vi "SSL Vision Log Player.vi"() -> ()   [LabVIEW 2016]
uses:
  SSL Detection Frame.ctl
  SSL Detection Robot.ctl
  SSL Detection Ball.ctl
  <extravilib>/ChannelInstances/Stream-a[.](u8)/Read With Abort.vi
  <extravilib>/ChannelInstances/Stream-a[.](u8)/Write With Abort.vi
  <extravilib>/ChannelInstances/Stream-a[.](u8)/Endpoint.vi
  <vilib>/Utility/tcp.llb/UDP Multicast Read-Only Open.vi
  <extravilib>/ChannelInstances/Stream-a[.](u8)/Instantiate.vi
  <extravilib>/ChannelInstances/Stream-a[.](u8)/)Channel.vi
  <resource>/ChannelSupport/_ChannelSupport/WaitIfNeeded.vi
  Varint Decoder uint64.vi
  Varint Decoder uint32.vi
  <extravilib>/ChannelInstances/Stream-a[.](u8).lvlib
panel:
  out "Varint 6":u64
  out "Varint 5":u32
  out "Varint 4":u64
  out "Varint 3":i32
  out "Varint 2":u64
  out "Varint":u64
  out "error out 3":errorcluster
  out "Boolean":bool
  out "Boolean 2":bool
  out "error out":errorcluster
  out "count 2":i32
  out "count":i32
  out "2D Picture":picture
  out "Detection Frame 2":T1 {"t_sent" format="%#_6f"; "t_capture" format="%#.6f"}
  in  "Modo":bool
  in  "Multicast Port:":u16=10020
  out "Data Read":i32 format="%.3p"
  out "Numeric":i32
  out "error out 2":errorcluster
  in  "file path (use dialog)":path=path "E:/Media/2016-07-01_cmdragons_immortals.log"
  in  "Multicast Address:":string="224.5.23.2"
  # "UDP"
  # "LOG"
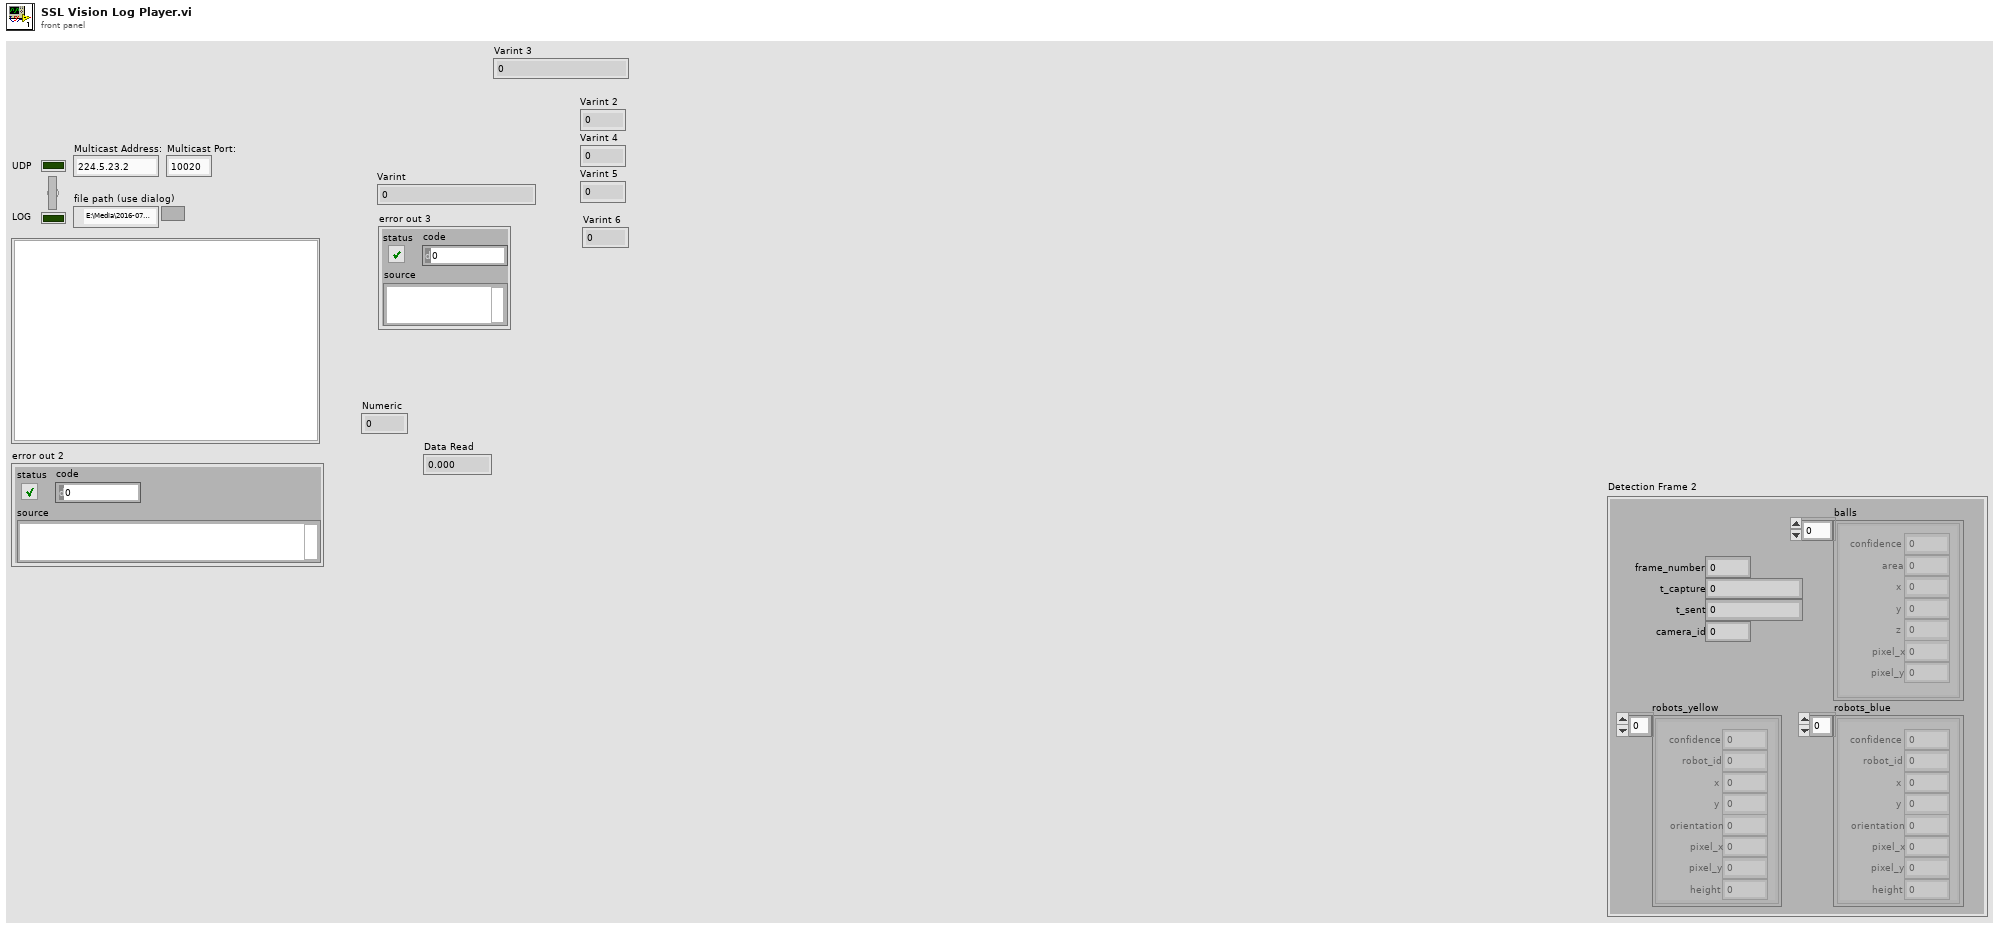
[diagram p1: front panel]
types:
  T1 = typedef "SSL Detection Frame.ctl" = cluster{"frame_number":u32, "t_capture":dbl, "t_sent":dbl, "camera_id":u32, "robots_yellow":T2[], "robots_blue":T2[], "balls":T3[]}
  T2 = typedef "SSL Detection Robot.ctl" = cluster{"x":dbl, "robot_id":u32, "confidence":sgl, "y":sgl, "orientation":sgl, "pixel_x":sgl, "pixel_y":sgl, "height":sgl}
  T3 = typedef "SSL Detection Ball.ctl" = cluster{"x":sgl, "area":u32, "confidence":sgl, "y":sgl, "z":sgl, "pixel_x":sgl, "pixel_y":sgl}
  T4 = enum16{"open", "replace", "create", "open or create", "replace or create", "replace or create with confirmation"}
  T5 = typedef "Stream-a[.](u8).lvlib/)Channel.ctl" = refnum<queue>
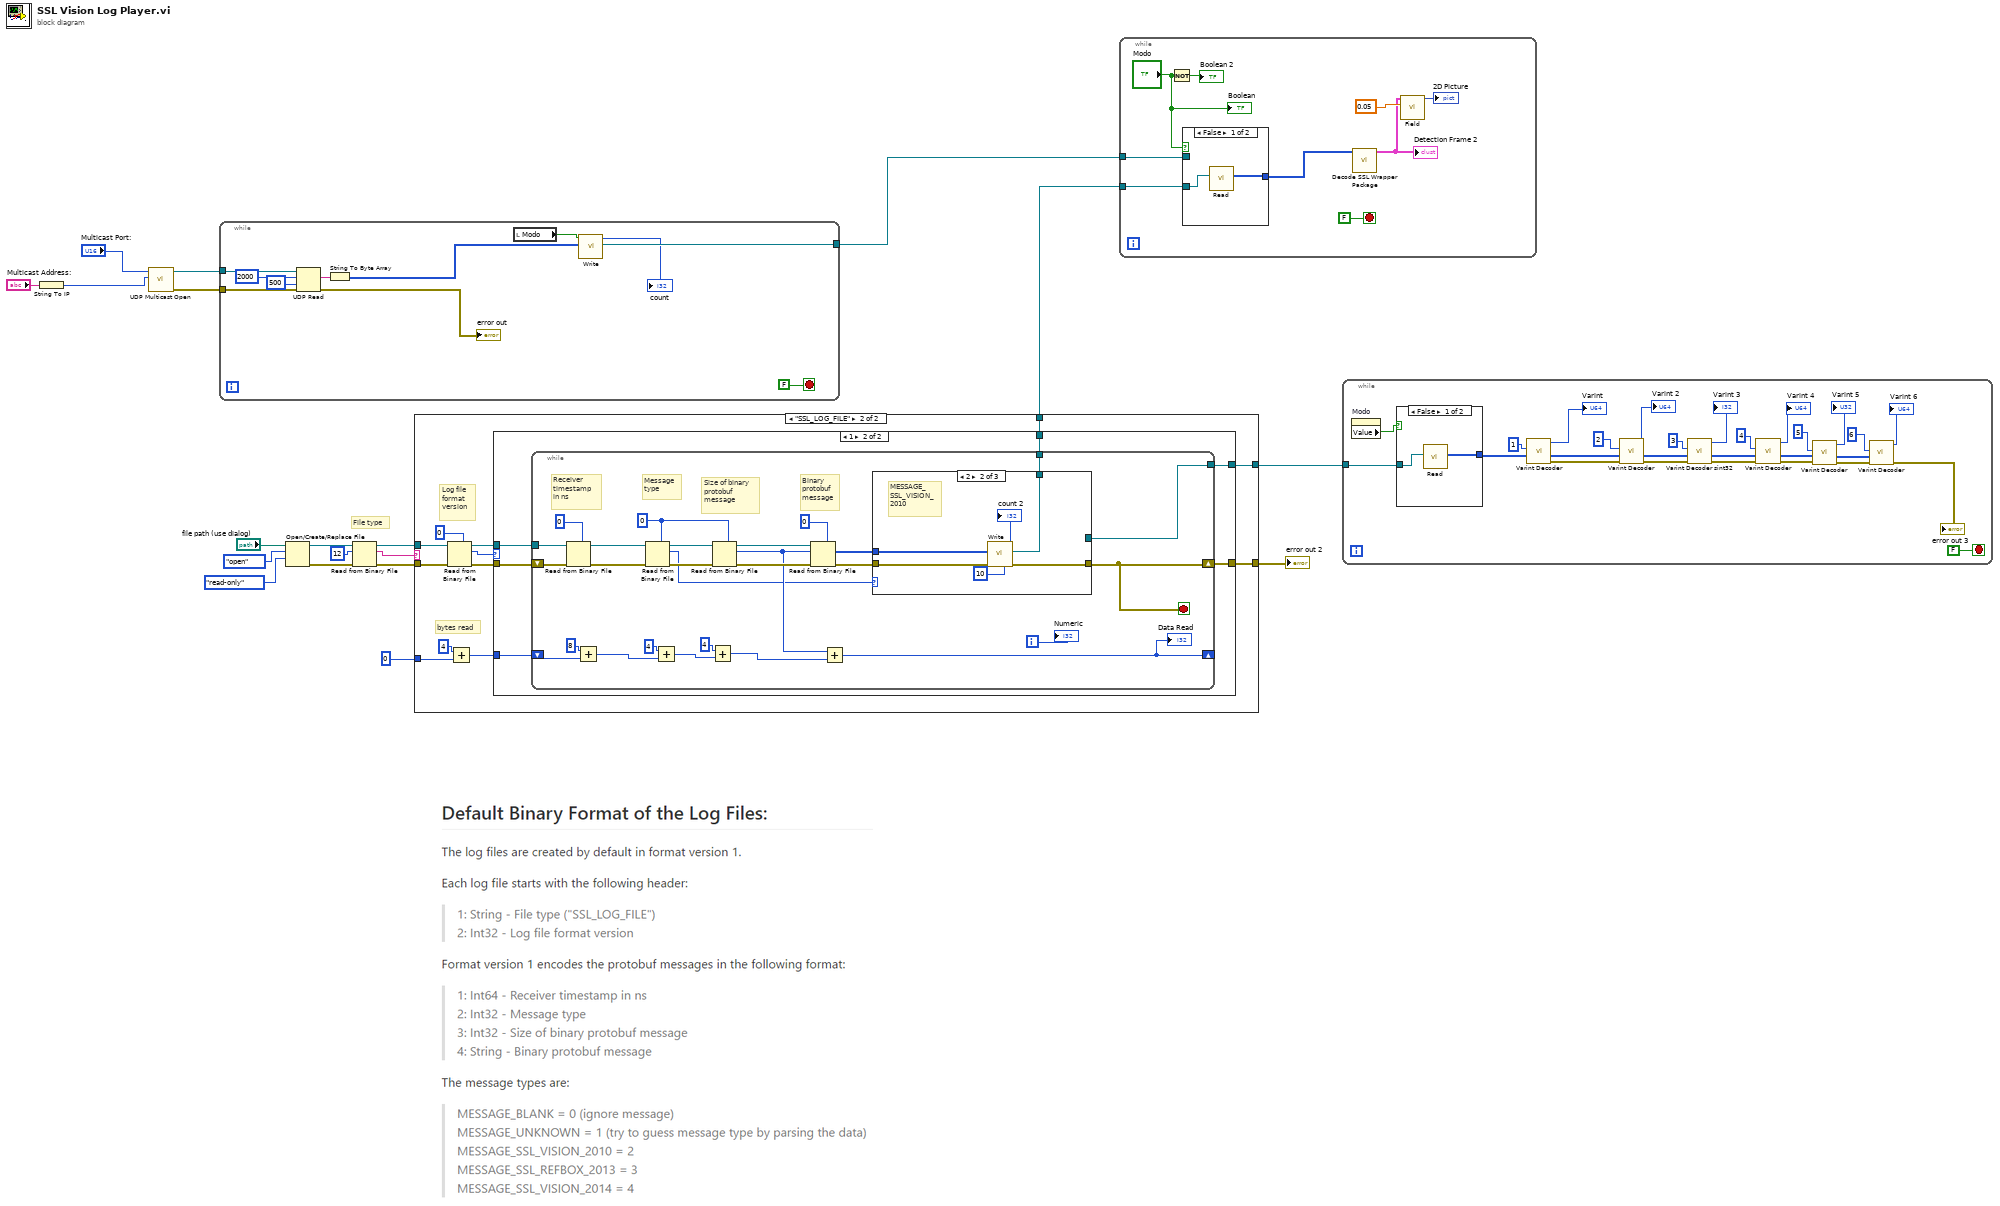
[diagram p0: block diagram]
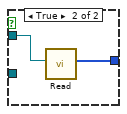
[diagram p3: hidden frame]
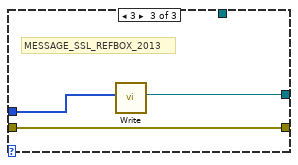
[diagram p7: hidden frame]
diagram:
  # "File type"
  n1 = String To IP(1:"Multicast Address:") -> (0:w18:u32)
  n2 = call-poly <vilib>:"UDP Multicast Open.vi"("multicast addr"=w18, "port"="Multicast Port:") -> ("error out"=w17:errorcluster, "connection ID"=w16:refnum<k16>)  [unwired: 7 in, 1 out]
  n3 = while {
    tunnel: w17 -> [w30]
    tunnel: w16 -> [w29]
    tunnel: [w24] -> w2
    stop <- FALSE stop-if-true
    n4 = UDP Read(connection ID=w29, max size (548)=2000, timeout ms (25000)=500, 8:w30) -> (data out=w28:string, error out=→"error out":errorcluster)  [unwired: 3 out]
    n5 = String To Byte Array(string=w28) -> (unsigned byte array=w25:u8[])
    n6 = local read "Modo"() -> (w21:bool)
    n7 = call <extravilib>:"Write.vi"("element"=w25, "element valid? (T)"=w21) -> ("channel"=w24:T5, "count"=→"count":i32)  [unwired: 7 in, 1 out]
  }
  n8 = Open/Create/Replace File(file path (use dialog)="file path (use dialog)", operation (0:open)=T4."open", access (0:read/write)=enum16{"read/write", "read-only", "write-only"}."read-only") -> (refnum out=w12:refnum<file>, error out=w13:errorcluster)  [unwired: 3 in, 1 out]
  n9 = Read from Binary File(8:w13, 10:12 ("count (1)"), 11:w12) -> (0:w9:errorcluster, 2:w7:string, 3:w10:refnum<file>)  [unwired: 3 in, 1 out]
  n10 = case shown="\"SSL_LOG_FILE\"" w7 {
    tunnel: w10 -> [_ w42]
    tunnel: w9 -> [w31 w41]
    tunnel: 0 -> [_ w38]
    tunnel: [w31 w34] -> w6
    tunnel: [_ w33] -> w3
    tunnel: [_ w32] -> w1
    frame Default {
    }
    frame "SSL_LOG_FILE" {
      # "bytes read"
      # "Log file \nformat \nversion"
      n11 = Read from Binary File(5:0 ("prompt (Open existing file)"), 8:w41, 11:w42) -> (0:w40:errorcluster, 2:w35:i32, 3:w39:refnum<file>)  [unwired: 3 in, 1 out]
      n12 = Add(x=4, y=w38) -> (x+y=w36:i32)
      n13 = case shown="1" w35 {
        tunnel: w39 -> [_ w50]
        tunnel: w40 -> [w44 w49]
        tunnel: w36 -> [_ w48]
        tunnel: [w44 w47] -> w34
        tunnel: [_ w46] -> w33
        tunnel: [_ w45] -> w32
        frame Default {
        }
        frame 1 {
          n14 = while {
            tunnel: w50 -> [w75]
            shift-right: [w53] -> w47
            shift-left: w49 -> [w74]
            shift-right: [w55] -> _
            shift-left: w48 -> [w62]
            tunnel: [w52] -> w46
            tunnel: [w51] -> w45
            i -> [w64]
            stop <- w53 stop-if-true
            w67 = 0 ("data type")
            # "Binary\nprotobuf\nmessage"
            # "Size of binary\nprotobuf \nmessage"
            # "Receiver \ntimestamp \nin ns"
            # "Message\ntype"
            n15 = Read from Binary File(5:i64 0 ("data type"), 8:w74, 11:w75) -> (0:w72:errorcluster, 3:w73:refnum<file>)  [unwired: 3 in, 2 out]
            n16 = Add(x=8, y=w62) -> (x+y=w60:i32)
            n17 = Read from Binary File(5:w67, 8:w72, 11:w73) -> (0:w69:errorcluster, 2:w54:i32, 3:w71:refnum<file>)  [unwired: 3 in, 1 out]
            n18 = Add(x=4, y=w60) -> (x+y=w58:i32)
            n19 = Add(x=4, y=w58) -> (x+y=w56:i32)
            n20 = Read from Binary File(5:w67, 8:w69, 11:w71) -> (0:w68:errorcluster, 2:w57:i32, 3:w70:refnum<file>)  [unwired: 3 in, 1 out]
            n21 = Read from Binary File(5:u8 0 ("data type"), 8:w68, 10:w57, 11:w70) -> (0:w65:errorcluster, 2:w66:u8[])  [unwired: 2 in, 2 out]
            n22 = Add(x=w57, y=w56) -> (x+y=w55:i32)
            "Data Read" <- w55
            n23 = case shown="2" w54 {
              tunnel: w66 -> [_ w83 w85]
              tunnel: w65 -> [w78 w82 w86]
              tunnel: [w78 w82 w86] -> w53
              tunnel: [_ w81 _] -> w52
              tunnel: [_ _ w84] -> w51
              frame Default {
              }
              frame 2 {
                # "MESSAGE_\nSSL_VISION_\n2010"
                n24 = call <extravilib>:"Write.vi"("size (unlimited)"=10, "element"=w83) -> ("channel"=w81:T5, "count"=→"count 2":i32)  [unwired: 7 in, 1 out]
              }
              frame 3 {
                # "MESSAGE_SSL_REFBOX_2013"
                n25 = call <extravilib>:"Write.vi"("element"=w85) -> ("channel"=w84:T5)  [unwired: 8 in, 2 out]
              }
            }
            "Numeric" <- w64
          }
        }
      }
    }
  }
  "error out 2" <- w6
  n26 = while {
    tunnel: w3 -> [w89]
    tunnel: w2 -> [w90]
    stop <- FALSE stop-if-true
    n27 = Not(x="Modo") -> (.not. x?=→"Boolean 2":bool)
    n28 = case shown="False" "Modo" {
      tunnel: [w97 w98] -> w91
      tunnel: w90 -> [_ w99]
      tunnel: w89 -> [w96 _]
      frame False {
        n29 = call <extravilib>:"Read.vi"("channel"=w96) -> ("element"=w97:u8[])  [unwired: 6 in, 4 out]
      }
      frame True {
        n30 = call <extravilib>:"Read.vi"("channel"=w99) -> ("element"=w98:u8[])  [unwired: 6 in, 4 out]
      }
    }
    n31 = call "Decode SSL Wrapper Package.vi"("unsigned byte array"=w91) -> ("Detection Frame"=w93:T1)  [unwired: 7 in, 3 out]
    "Detection Frame 2" <- w93
    n32 = call "Field.vi"("Scale mm/pixel"=0.05, "Detection Frame"=w93) -> ("2D Picture"=→"2D Picture":picture)  [unwired: 9 in]
    "Boolean" <- "Modo"
  }
  n33 = while {
    tunnel: w1 -> [w126]
    stop <- FALSE stop-if-true
    n34 = property on="Modo" class="Bool (strict)"() -> ("Value"=w125:bool)  [unwired: 2 in, 2 out]
    n35 = case shown="False" w125 {
      tunnel: [w128 _] -> w123
      tunnel: w126 -> [w127 _]
      frame False {
        n36 = call <extravilib>:"Read.vi"("channel"=w127) -> ("element"=w128:u8[])  [unwired: 6 in, 4 out]
      }
      frame True {
      }
    }
    n37 = call-poly "Varint Decoder.vi"("Array"=w123, "Key"=1) -> ("error out"=w120:errorcluster, "array w/ subset deleted"=w119:u8[], "Varint"=→"Varint":u64)  [unwired: 6 in, 1 out]
    n38 = call-poly "Varint Decoder.vi"("error in (no error)"=w120, "Array"=w119, "Key"=2) -> ("error out"=w116:errorcluster, "array w/ subset deleted"=w114:u8[], "Varint"=→"Varint 2":u64)  [unwired: 5 in, 1 out]
    n39 = call "Varint Decoder sint32.vi"("error in (no error)"=w116, "Array"=w114, "Key"=3) -> ("error out"=w112:errorcluster, "array w/ subset deleted"=w111:u8[], "Varint"=→"Varint 3":i32)  [unwired: 5 in, 1 out]
    n40 = call-poly "Varint Decoder.vi"("error in (no error)"=w112, "Array"=w111, "Key"=4) -> ("error out"=w108:errorcluster, "array w/ subset deleted"=w106:u8[], "Varint"=→"Varint 4":u64)  [unwired: 5 in, 1 out]
    n41 = call-poly "Varint Decoder.vi"("error in (no error)"=w108, "Array"=w106, "Key"=5) -> ("error out"=w107:errorcluster, "array w/ subset deleted"=w105:u8[], "Varint"=→"Varint 5":u32)  [unwired: 5 in, 1 out]
    n42 = call-poly "Varint Decoder.vi"("error in (no error)"=w107, "Array"=w105, "Key"=6) -> ("error out"=→"error out 3":errorcluster, "Varint"=→"Varint 6":u64)  [unwired: 5 in, 2 out]
  }
